vi "2_HelloUser.vi"() -> ()   [LabVIEW 2015]
panel:
  out "Greeting":string
  in  "Enter your name":string
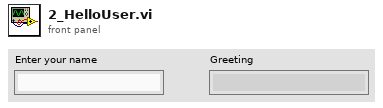
[diagram p1: front panel]
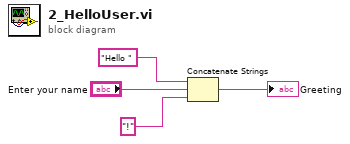
[diagram p0: block diagram]
diagram:
  n1 = Concatenate Strings("Hello " ("string"), "Enter your name", "!" ("string")) -> (→"Greeting":string)
